vi "make_terminals.vi"(10 "GObj引用句柄":refnum<vi>, 11 "node_type":string) -> (3 "terminals_out":T1[](array[typedef]))   [LabVIEW 2020]
uses:
  terminalData.ctl
  terminal_type.ctl
  terminal_direction.ctl
panel:
  out "大小 6":i32
  out "大小 5":i32
  out "大小 4":i32
  out "大小 3":i32
  out "大小 2":i32
  out "大小":i32
  # "tunnel/judge/shift?"
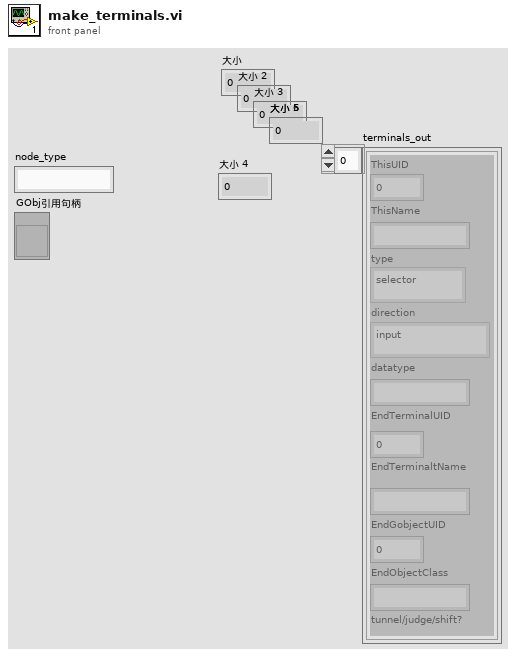
[diagram p1: front panel]
types:
  T1 = typedef "terminalData.ctl" = cluster{"ThisUID":i32, "ThisName":string, "type":T2, "direction":T3, "datatype":string, "EndTerminalUID":i32, "EndTerminaltName":string, "EndGobjectUID":i32, "EndObjectClass":string}
  T2 = typedef "terminal_type.ctl" = enum16{"selector", "tunnel", "shift", "timeout", "normal", "floating"}
  T3 = typedef "terminal_direction.ctl" = enum16{"input", "output"}
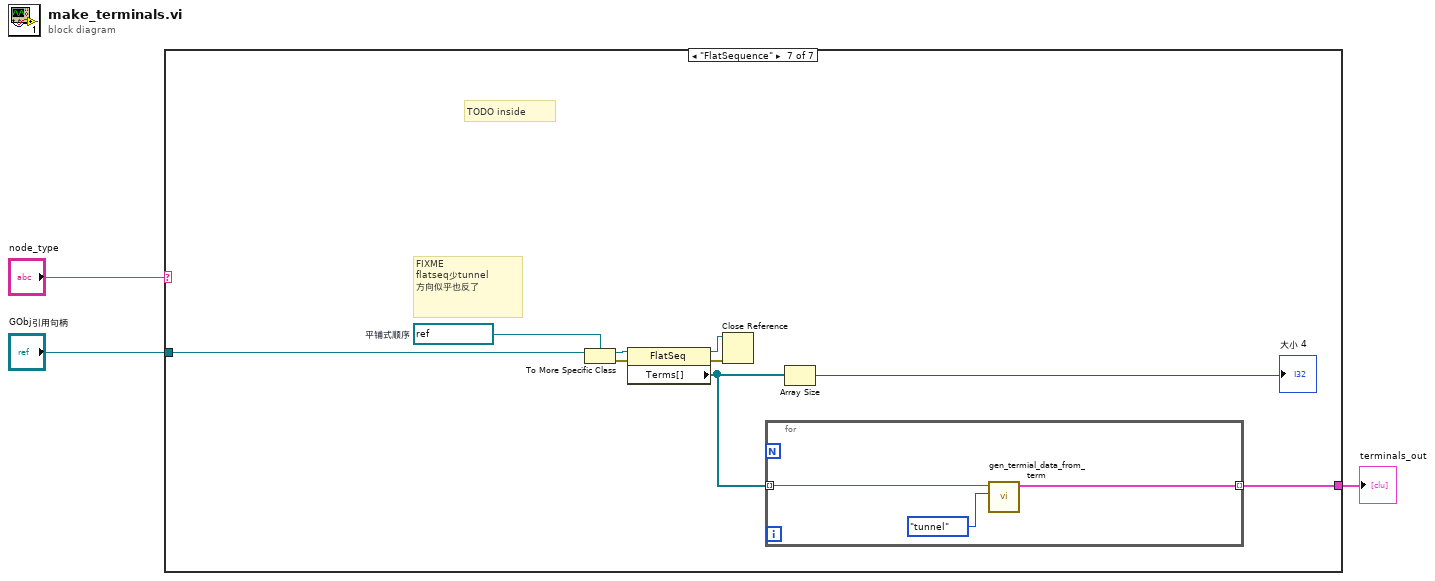
[diagram p0: block diagram]
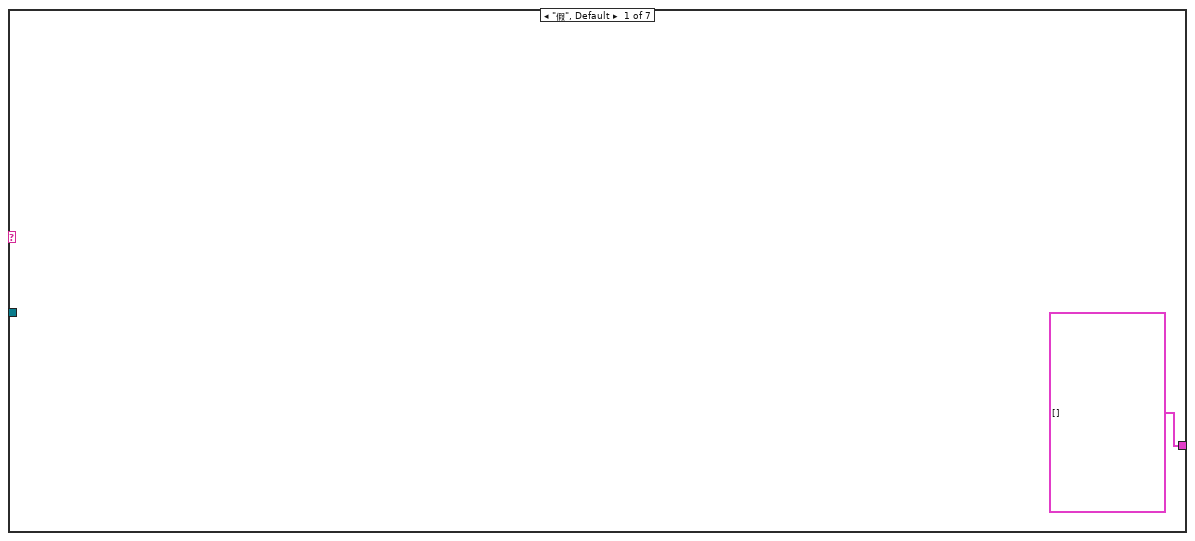
[diagram p2: hidden frame]
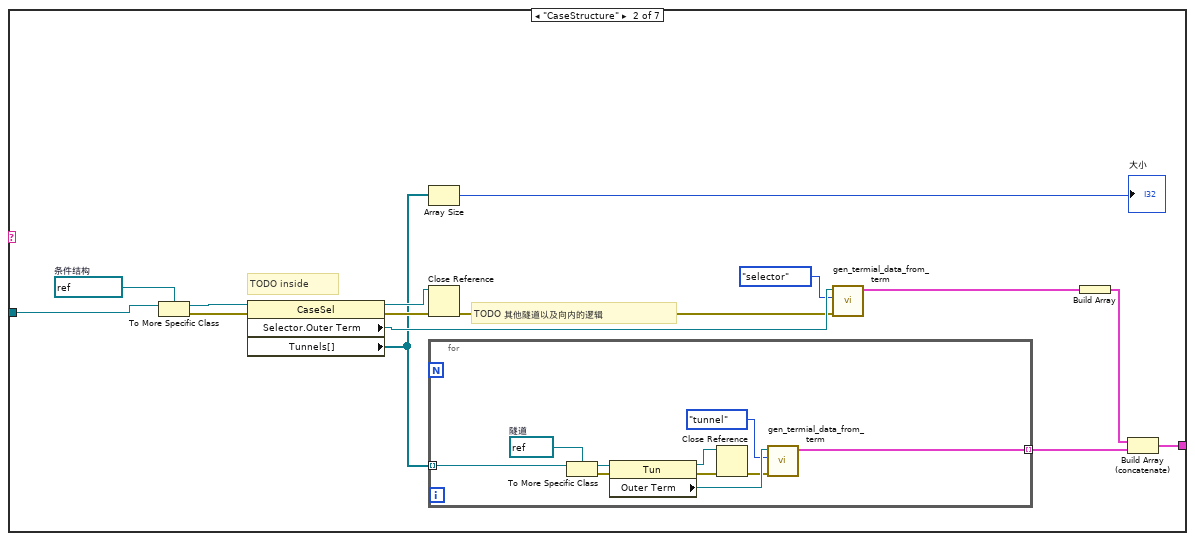
[diagram p3: hidden frame]
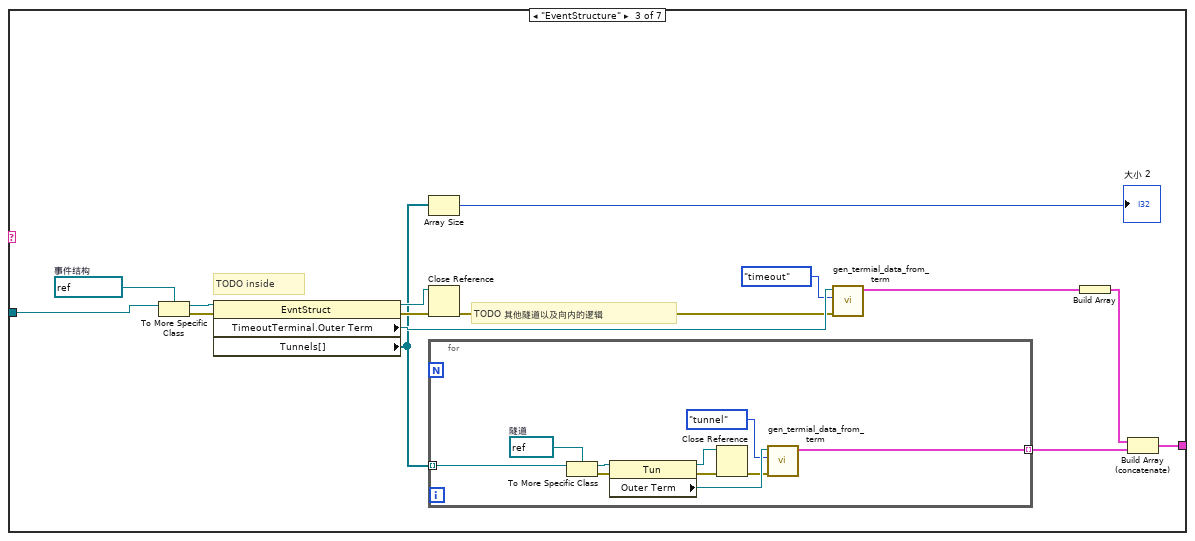
[diagram p4: hidden frame]
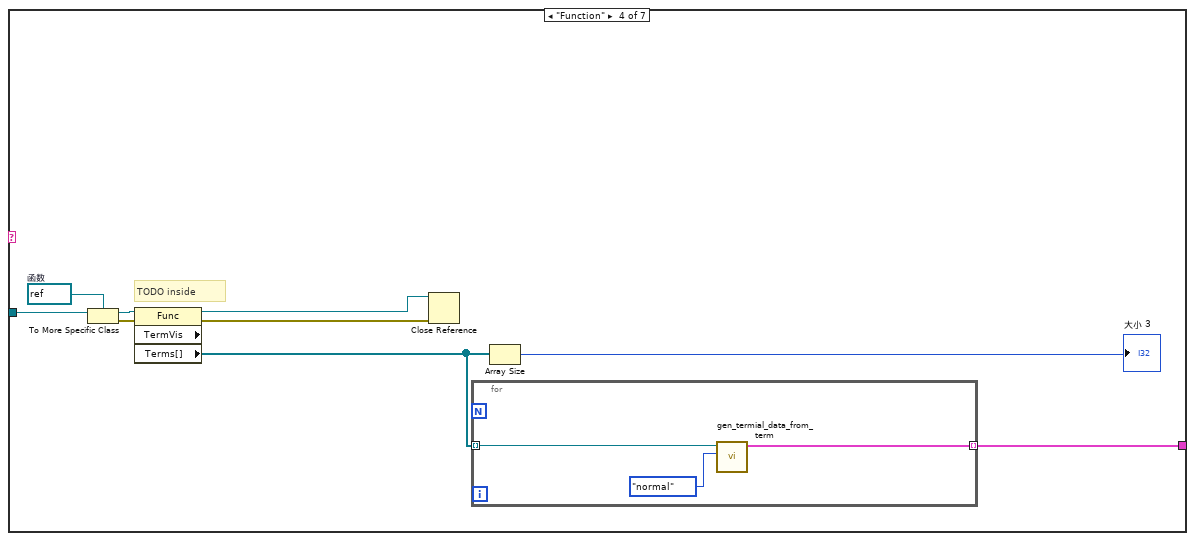
[diagram p5: hidden frame]
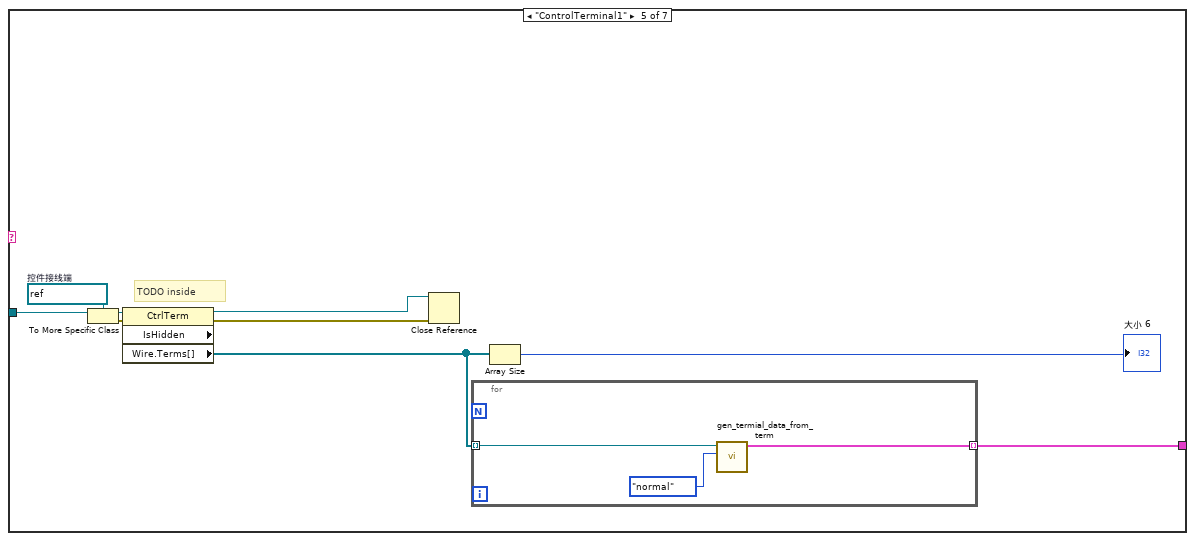
[diagram p6: hidden frame]
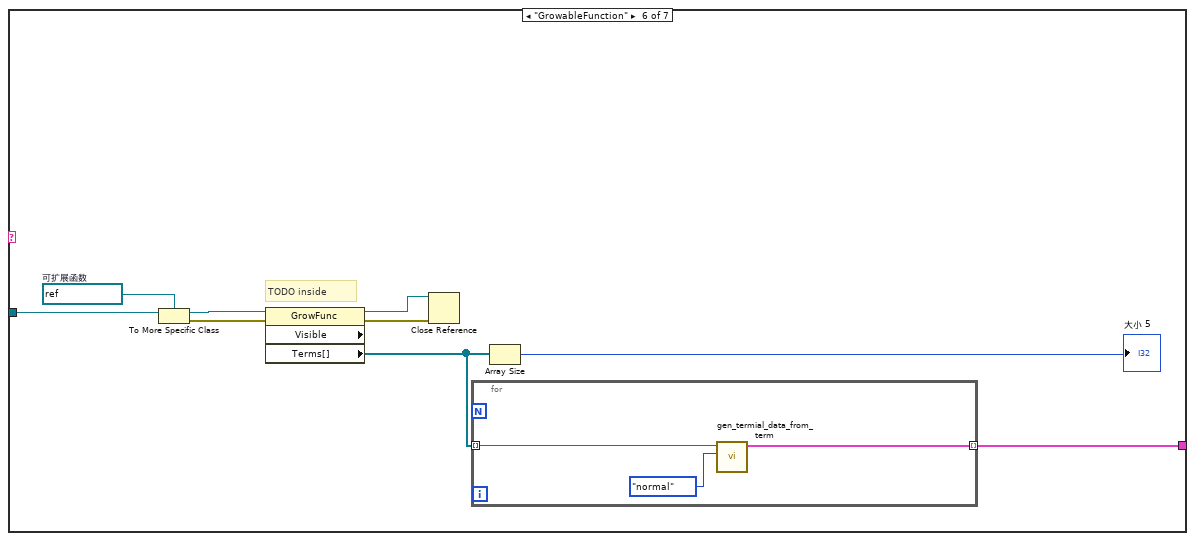
[diagram p7: hidden frame]
diagram:
  n1 = case shown="\"FlatSequence\"" "node_type" {
    tunnel: "GObj引用句柄" -> [_ w16 w41 w60 w72 w84 w96]
    tunnel: [T1[] [] w5 w30 w55 w67 w79 w91] -> w1
    frame "假", Default {
    }
    frame "CaseStructure" {
      w17 = refnum<vi> refnum  # 条件结构
      # "TODO 其他隧道以及向内的逻辑"
      # "TODO inside"
      n2 = To More Specific Class ("转换为特定的类")(target class=w17, reference=w16) -> (specific class reference=w19:refnum<vi>, error out=w18:errorcluster)  [unwired: 1 in]
      n3 = property on="属性节点" class="CaseSel"(reference=w19, error in=w18) -> (reference out=w15:refnum<vi>, error out=w14:errorcluster, "Selector.Outer Term"=w13:refnum<vi>, "Tunnels[]"=w9:refnum<vi>[])
      n4 = Array Size ("数组大小")(array=w9) -> (size(s)=→"大小":i32)
      n5 = Close Reference ("关闭引用")(reference=w15, error in (no error)=w14) -> (error out=w12:errorcluster)
      n6 = for {
        tunnel: w9 -> [w27] mode=indexing
        tunnel: [w20] -> w6 mode=indexing
        w29 = refnum<vi> refnum  # 隧道
        n7 = To More Specific Class ("转换为特定的类")(target class=w29, reference=w27) -> (specific class reference=w28:refnum<vi>, error out=w24:errorcluster)  [unwired: 1 in]
        n8 = property on="属性节点" class="Tun"(reference=w28, error in=w24) -> (reference out=w26:refnum<vi>, error out=w25:errorcluster, "Outer Term"=w23:refnum<vi>)
        n9 = Close Reference ("关闭引用")(reference=w26, error in (no error)=w25) -> (error out=w22:errorcluster)
        n10 = call "gen_termial_data_from_term.vi"("错误输入（无错误）"=w22, "type"=terminal_type."tunnel", "Term引用句柄"=w23) -> ("terminal"=w20:T1)  [unwired: 8 in]
      }
      n11 = call "gen_termial_data_from_term.vi"("错误输入（无错误）"=w12, "type"=terminal_type."selector", "Term引用句柄"=w13) -> ("terminal"=w11:T1)  [unwired: 8 in]
      n12 = Build Array ("创建数组")(w11) -> (w7:T1[])
      n13 = Build Array (concatenate) ("创建数组")(w7, w6) -> (w5:T1[])
    }
    frame "EventStructure" {
      w42 = refnum<vi> refnum  # 事件结构
      # "TODO 其他隧道以及向内的逻辑"
      # "TODO inside"
      n14 = To More Specific Class ("转换为特定的类")(target class=w42, reference=w41) -> (specific class reference=w44:refnum<vi>, error out=w43:errorcluster)  [unwired: 1 in]
      n15 = property on="属性节点" class="EvntStruct"(reference=w44, error in=w43) -> (reference out=w40:refnum<vi>, error out=w39:errorcluster, "TimeoutTerminal.Outer Term"=w38:refnum<vi>, "Tunnels[]"=w34:refnum<vi>[])
      n16 = Array Size ("数组大小")(array=w34) -> (size(s)=→"大小 2":i32)
      n17 = Close Reference ("关闭引用")(reference=w40, error in (no error)=w39) -> (error out=w37:errorcluster)
      n18 = for {
        tunnel: w34 -> [w52] mode=indexing
        tunnel: [w45] -> w31 mode=indexing
        w54 = refnum<vi> refnum  # 隧道
        n19 = To More Specific Class ("转换为特定的类")(target class=w54, reference=w52) -> (specific class reference=w53:refnum<vi>, error out=w49:errorcluster)  [unwired: 1 in]
        n20 = property on="属性节点" class="Tun"(reference=w53, error in=w49) -> (reference out=w51:refnum<vi>, error out=w50:errorcluster, "Outer Term"=w48:refnum<vi>)
        n21 = Close Reference ("关闭引用")(reference=w51, error in (no error)=w50) -> (error out=w47:errorcluster)
        n22 = call "gen_termial_data_from_term.vi"("错误输入（无错误）"=w47, "type"=terminal_type."tunnel", "Term引用句柄"=w48) -> ("terminal"=w45:T1)  [unwired: 8 in]
      }
      n23 = call "gen_termial_data_from_term.vi"("错误输入（无错误）"=w37, "type"=terminal_type."timeout", "Term引用句柄"=w38) -> ("terminal"=w36:T1)  [unwired: 8 in]
      n24 = Build Array ("创建数组")(w36) -> (w32:T1[])
      n25 = Build Array (concatenate) ("创建数组")(w32, w31) -> (w30:T1[])
    }
    frame "Function" {
      w61 = refnum<vi> refnum  # 函数
      # "TODO inside"
      n26 = To More Specific Class ("转换为特定的类")(target class=w61, reference=w60) -> (specific class reference=w63:refnum<vi>, error out=w62:errorcluster)  [unwired: 1 in]
      n27 = property on="属性节点" class="Func" props=["TermVis", "Terms[]"](reference=w63, error in=w62) -> (reference out=w59:refnum<vi>, error out=w58:errorcluster, "Terms[]"=w56:refnum<vi>[])  [unwired: 1 out]
      n28 = Close Reference ("关闭引用")(reference=w59, error in (no error)=w58) -> ()  [unwired: 1 out]
      n29 = for {
        tunnel: w56 -> [w64] mode=indexing
        tunnel: [w65] -> w55 mode=indexing
        n30 = call "gen_termial_data_from_term.vi"("type"=terminal_type."normal", "Term引用句柄"=w64) -> ("terminal"=w65:T1)  [unwired: 9 in]
      }
      n31 = Array Size ("数组大小")(array=w56) -> (size(s)=→"大小 3":i32)
    }
    frame "ControlTerminal1" {
      w73 = refnum<vi> refnum  # 控件接线端
      # "TODO inside"
      n32 = To More Specific Class ("转换为特定的类")(target class=w73, reference=w72) -> (specific class reference=w75:refnum<vi>, error out=w74:errorcluster)  [unwired: 1 in]
      n33 = property on="属性节点" class="CtrlTerm" props=["IsHidden", "Wire", "Terms[]"](reference=w75, error in=w74) -> (reference out=w71:refnum<vi>, error out=w70:errorcluster, "Wire.Terms[]"=w68:refnum<vi>[])  [unwired: 1 out]
      n34 = Close Reference ("关闭引用")(reference=w71, error in (no error)=w70) -> ()  [unwired: 1 out]
      n35 = for {
        tunnel: w68 -> [w76] mode=indexing
        tunnel: [w77] -> w67 mode=indexing
        n36 = call "gen_termial_data_from_term.vi"("type"=terminal_type."normal", "Term引用句柄"=w76) -> ("terminal"=w77:T1)  [unwired: 9 in]
      }
      n37 = Array Size ("数组大小")(array=w68) -> (size(s)=→"大小 6":i32)
    }
    frame "GrowableFunction" {
      w85 = refnum<vi> refnum  # 可扩展函数
      # "TODO inside"
      n38 = To More Specific Class ("转换为特定的类")(target class=w85, reference=w84) -> (specific class reference=w87:refnum<vi>, error out=w86:errorcluster)  [unwired: 1 in]
      n39 = property on="属性节点" class="GrowFunc" props=["Visible", "Terms[]"](reference=w87, error in=w86) -> (reference out=w83:refnum<vi>, error out=w82:errorcluster, "Terms[]"=w80:refnum<vi>[])  [unwired: 1 out]
      n40 = Close Reference ("关闭引用")(reference=w83, error in (no error)=w82) -> ()  [unwired: 1 out]
      n41 = for {
        tunnel: w80 -> [w88] mode=indexing
        tunnel: [w89] -> w79 mode=indexing
        n42 = call "gen_termial_data_from_term.vi"("type"=terminal_type."normal", "Term引用句柄"=w88) -> ("terminal"=w89:T1)  [unwired: 9 in]
      }
      n43 = Array Size ("数组大小")(array=w80) -> (size(s)=→"大小 5":i32)
    }
    frame "FlatSequence" {
      w97 = refnum<vi> refnum  # 平铺式顺序
      # "FIXME\nflatseq少tunnel\n方向似乎也反了"
      # "TODO inside"
      n44 = To More Specific Class ("转换为特定的类")(target class=w97, reference=w96) -> (specific class reference=w99:refnum<vi>, error out=w98:errorcluster)  [unwired: 1 in]
      n45 = property on="属性节点" class="FlatSeq"(reference=w99, error in=w98) -> (reference out=w95:refnum<vi>, error out=w94:errorcluster, "Terms[]"=w92:refnum<vi>[])
      n46 = Close Reference ("关闭引用")(reference=w95, error in (no error)=w94) -> ()  [unwired: 1 out]
      n47 = for {
        tunnel: w92 -> [w100] mode=indexing
        tunnel: [w101] -> w91 mode=indexing
        n48 = call "gen_termial_data_from_term.vi"("type"=terminal_type."tunnel", "Term引用句柄"=w100) -> ("terminal"=w101:T1)  [unwired: 9 in]
      }
      n49 = Array Size ("数组大小")(array=w92) -> (size(s)=→"大小 4":i32)
    }
  }
  "terminals_out" <- w1
